vi "Actor Core.vi"(8 "error in":errorcluster, 11 "Channel Scanner in":refnum<class "Channel Scanner.lvclass">) -> (0 "error out":errorcluster, 3 "Actor out":refnum<class "Actor.lvclass">)   [LabVIEW 2015, in "Channel Scanner.lvclass"]
doc: "(<B>Filename</B>: Actor Framework.lvlib:Actor.lvclass:Actor Core.vi)\n\nReceives messages to the actor, reacts to them, and initiates any error handling that may shut the actor down.\n\nDescendant classes may override this VI to append parallel tasks for the actor to complete while it handles messages. Overrides use the Call Parent Method node."
uses:
  Channel Scanner.lvclass
  <vilib>/ActorFramework/Actor/Actor.lvclass
  Channel Scanner Configuration.ctl
  Measure_core/Instrument Recorders/Instrument Recorder/Instrument Recorder.lvclass
panel:
  out "Name":string
  in  "Configuration":T1
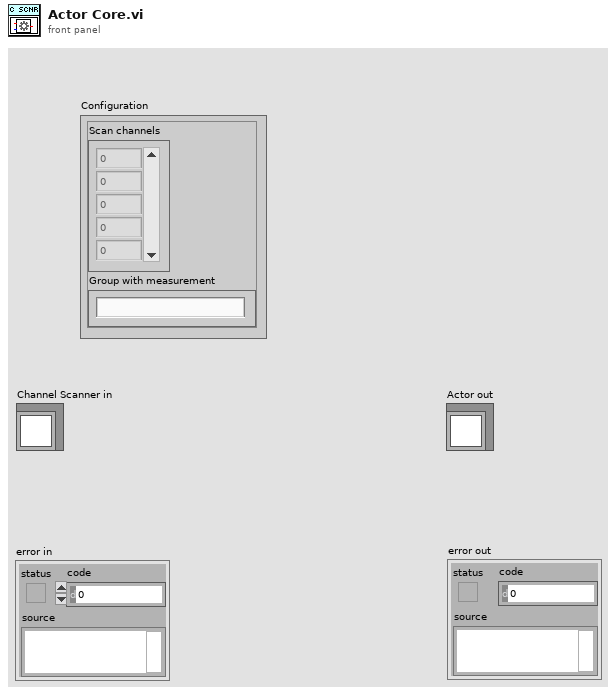
[diagram p1: front panel]
types:
  T1 = typedef "Channel Scanner Configuration.ctl" = cluster{"Scan channels":i32[], "Group with measurement":string}
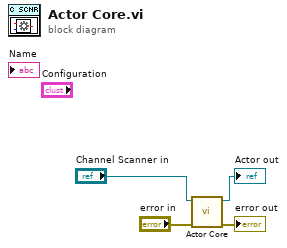
[diagram p0: block diagram]
diagram:
  n1 = call-parent "Actor Core.vi"("error in"="error in", "Measure Object in"="Channel Scanner in") -> ("error out"=→"error out":errorcluster, "Actor out"=→"Actor out":refnum<class "Actor.lvclass">)  [unwired: 8 in]
